vi "Take Portion of Data (single).vi"(8 "error in (no error)":errorcluster, 9 "Method":enum16{"Slider (%)", "X[] min and max"}(ring), 10 "Slider":cluster{dbl, dbl}(slide)={0.0, 0.5348837209302325} caption="Horizontal Slider" scale=0.0..1.0, 11 "XY-data in":cluster{"X-array":dbl[], "Y-array":dbl[]}) -> (0 "error out":errorcluster, 3 "XY-data out":cluster{"X-array":dbl[], "Y-array":dbl[]} {"Y-array" format="%.2p"; "X-array" format="%.2p"})   [LabVIEW 2016, in "xy_utilities.lvlib"]
uses:
  xy_utilities.lvlib
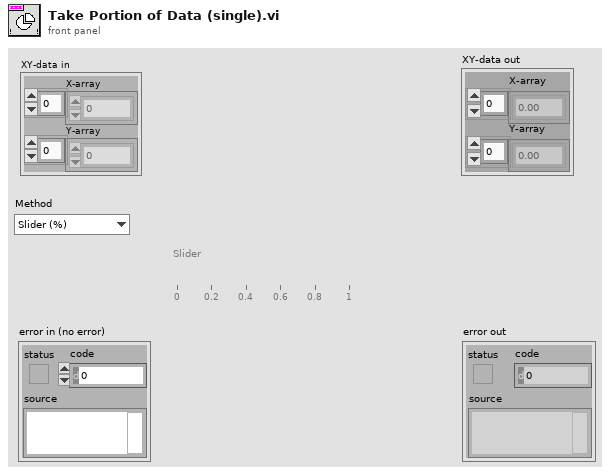
[diagram p1: front panel]
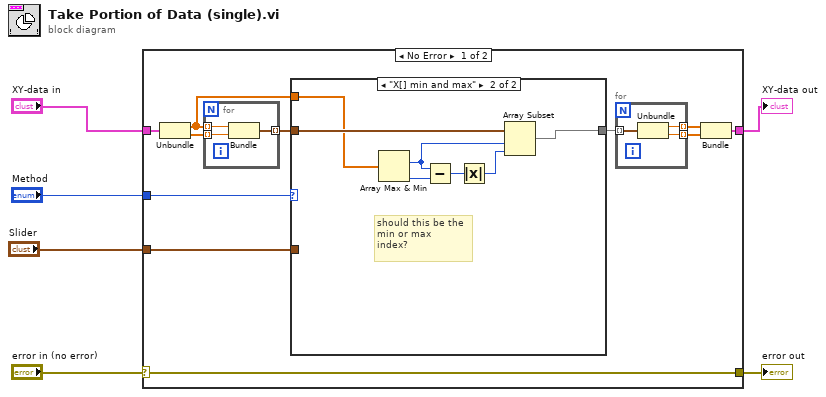
[diagram p0: block diagram]
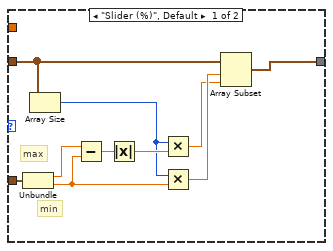
[diagram p2: hidden frame]
diagram:
  n1 = case shown="No Error" "error in (no error)" {
    selector: "error in (no error)" -> [w17 w42]
    tunnel: [w17 w42] -> w5
    tunnel: "XY-data in" -> [w16 w41]
    tunnel: [w9 w41] -> w3
    tunnel: "Method" -> [w13 _]
    tunnel: "Slider" -> [w8 _]
    frame No Error {
      n2 = Unbundle(w16) -> ("X-array"=w7:dbl[], "Y-array"=w15:dbl[])
      n3 = for {
        tunnel: w7 -> [w40] mode=indexing
        tunnel: w15 -> [w39] mode=indexing
        tunnel: [w38] -> w14 mode=indexing
        n4 = Bundle("x"=w40, "y"=w39) -> (w38:cluster{"x":dbl, "y":dbl})  [unwired: 1 in]
      }
      n5 = case shown="\"X[] min and max\"" w13 {
        tunnel: w14 -> [w24 w34]
        tunnel: [w23 w33] -> w10
        tunnel: w8 -> [w21 _]
        tunnel: w7 -> [_ w32]
        frame "Slider (%)", Default {
          # "min"
          # "max"
          n6 = Unbundle(w21) -> (w25:dbl, w22:dbl)
          n7 = Array Size(array=w24) -> (size(s)=w27:i32)
          n8 = Subtract(x=w25, y=w22) -> (x-y=w26:dbl)
          n9 = Absolute Value(x=w26) -> (abs(x)=w28:dbl)
          n10 = Multiply(x=w27, y=w28) -> (x*y=w29:dbl)
          n11 = Multiply(x=w27, y=w22) -> (x*y=w30:dbl)
          n12 = Array Subset(array=w24, index=w30, length=w29) -> (w23:cluster{"x":dbl, "y":dbl}[])
        }
        frame "X[] min and max" {
          # "should this be the\nmin or max\nindex?"
          n13 = Array Max & Min(array=w32) -> (max index (indices)=w31:i32, min index (indices)=w35:i32)  [unwired: 2 out]
          n14 = Subtract(x=w31, y=w35) -> (x-y=w36:i32)
          n15 = Absolute Value(x=w36) -> (abs(x)=w37:i32)
          n16 = Array Subset(array=w34, index=w31, length=w37) -> (w33:cluster{"x":dbl, "y":dbl}[])
        }
      }
      n17 = for {
        tunnel: w10 -> [w20] mode=indexing
        tunnel: [w19] -> w11 mode=indexing
        tunnel: [w18] -> w12 mode=indexing
        n18 = Unbundle(w20) -> ("x"=w19:dbl, "y"=w18:dbl)
      }
      n19 = Bundle(w11, w12) -> (w9:cluster{dbl[], dbl[]})  [unwired: 1 in]
    }
    frame Error {
    }
  }
  "error out" <- w5
  "XY-data out" <- w3
